vi "New Front Leg.vi"(9 "Leg up":bool, 10 "Command":enum16{"Down Closed", "Down Opened", "Up"}(ring), 11 "Old State":string) -> (1 "Claw":T1=enum."On", 2 "Foot":T1=enum."On", 3 "New state":string)   [LabVIEW 2012]
uses:
  <vilib>/Rock Robotics/WPI/Solenoid/WPI_SolenoidValue.ctl
  <vilib>/Rock Robotics/WPI/DriverStation/DriverStationLCD/WPI_DriverStationLCDLCDLine.ctl
panel:
  # "Be sure that \"Preallocated clone reentrant execution\"\nis checked in the VI Properties > Execution settings.\n(Right-click on the VI icon in the upper right to get to\nthe VI Properties window.)\n\nOne instance of the VI is used for the front leg and\none instance of the VI is used for the middle leg.\nThese instances must run independently or the \ntiming of the leg operations during the climb will be\nwrong."
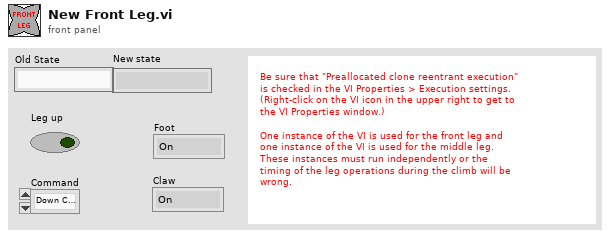
[diagram p1: front panel]
types:
  T1 = typedef "WPI_SolenoidValue.ctl" = enum16{"Off", "On", "Forward", "Reverse"}
  T2 = typedef "WPI_DriverStationLCDLCDLine.ctl" = enum16{"Main - Line 1", "User - Line 2", "User - Line 3", "User - Line 4", "User - Line 5", "User - Line 6"}
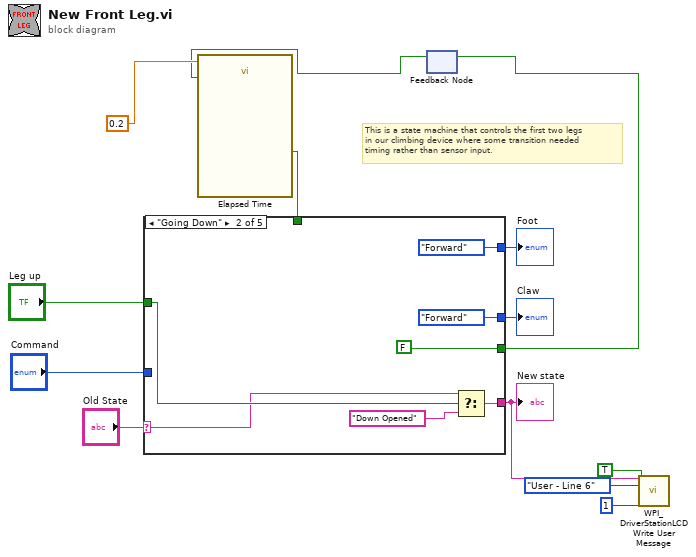
[diagram p0: block diagram]
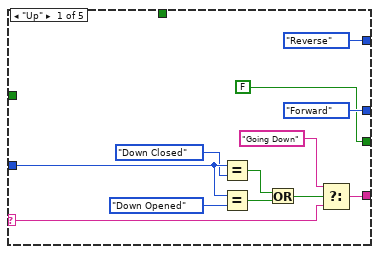
[diagram p2: hidden frame]
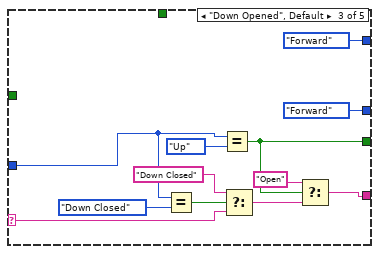
[diagram p3: hidden frame]
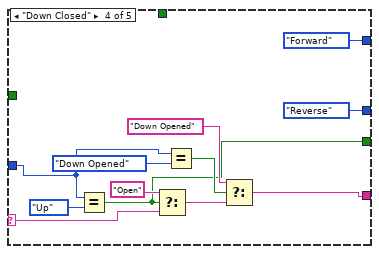
[diagram p4: hidden frame]
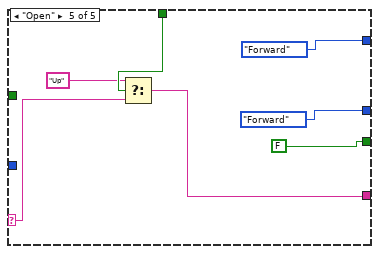
[diagram p5: hidden frame]
diagram:
  # "This is a state machine that controls the first two legs\nin our climbing device where some transition needed\ntiming rather than sensor input."
  n1 = feedback #1() -> (w7:bool)  [unwired: 1 in]
  n2 = call "Elapsed Time"("Time Target (s)"=0.2, "Reset"=w7) -> ("Time has Elapsed"=w5:bool)  [unwired: 10 in, 7 out]
  n3 = case shown="\"Going Down\"" "Old State" {
    selector: "Old State" -> [w21 w27 w43 w52 w59]
    tunnel: [WPI_SolenoidValue."Forward" ("Foot") WPI_SolenoidValue."Forward" ("Foot") WPI_SolenoidValue."Forward" ("Foot") WPI_SolenoidValue."Reverse" ("Foot") WPI_SolenoidValue."Forward" ("Foot")] -> w13
    tunnel: [w23 w30 w34 w46 w61] -> w4
    tunnel: [WPI_SolenoidValue."Reverse" ("Foot") WPI_SolenoidValue."Forward" ("Foot") WPI_SolenoidValue."Forward" ("Foot") WPI_SolenoidValue."Forward" ("Foot") WPI_SolenoidValue."Forward" ("Foot")] -> w12
    tunnel: "Leg up" -> [_ w29 _ _ _]
    tunnel: "Command" -> [w19 _ w36 w50 _]
    tunnel: [FALSE ("Time has Elapsed") FALSE ("Time has Elapsed") w33 w45 FALSE ("Time has Elapsed")] -> w6
    tunnel: w5 -> [_ _ _ _ w62]
    frame "Up" {
      n4 = Equal?(x=w19, y=enum16{"Down Closed", "Down Opened", "Up"}."Down Closed") -> (x = y?=w16:bool)
      n5 = Equal?(x=w19, y=enum16{"Down Closed", "Down Opened", "Up"}."Down Opened") -> (x = y?=w17:bool)
      n6 = Or(x=w16, y=w17) -> (x .or. y?=w15:bool)
      n7 = Select(t="Going Down" ("f"), s=w15, f=w21) -> (s? t:f=w23:string)
    }
    frame "Going Down" {
      n8 = Select(t=w27, s=w29, f="Down Opened" ("t")) -> (s? t:f=w30:string)
    }
    frame "Down Opened", Default {
      n9 = Equal?(x=w36, y=enum16{"Down Closed", "Down Opened", "Up"}."Down Closed") -> (x = y?=w39:bool)
      n10 = Equal?(x=w36, y=enum16{"Down Closed", "Down Opened", "Up"}."Up") -> (x = y?=w33:bool)
      n11 = Select(t="Down Closed", s=w39, f=w43) -> (s? t:f=w38:string)
      n12 = Select(t="Open", s=w33, f=w38) -> (s? t:f=w34:string)
    }
    frame "Down Closed" {
      n13 = Equal?(x=w50, y=enum16{"Down Closed", "Down Opened", "Up"}."Up") -> (x = y?=w45:bool)
      n14 = Select(t="Open", s=w45, f=w52) -> (s? t:f=w51:string)
      n15 = Equal?(x=w50, y=enum16{"Down Closed", "Down Opened", "Up"}."Down Opened") -> (x = y?=w48:bool)
      n16 = Select(t="Down Opened", s=w48, f=w51) -> (s? t:f=w46:string)
    }
    frame "Open" {
      n17 = Select(t="Up", s=w62, f=w59) -> (s? t:f=w61:string)
    }
  }
  "Foot" <- w12
  "Claw" <- w13
  "New state" <- w4
  n18 = feedback-in #1(w6) -> ()
  n19 = call <vilib>:"WPI_DriverStationLCDWrite User Message.vi"("line text"=w4, "line"=WPI_DriverStationLCDLCDLine."User - Line 6", "starting column"=i8 1, "clear line before write (T)"=TRUE) -> ()  [unwired: 11 in, 1 out]
